vi "HW operation 3.vi"(1 "stop":bool) -> (0 "Numeric":dbl)   [LabVIEW 2018]
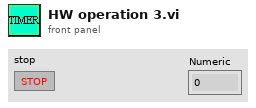
[diagram p1: front panel]
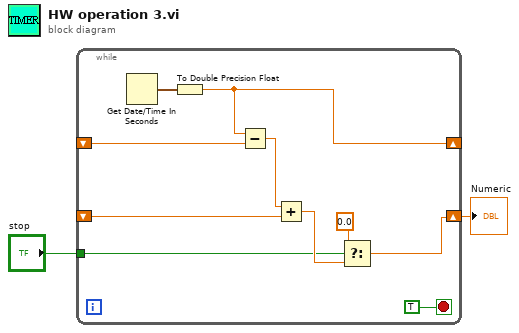
[diagram p0: block diagram]
diagram:
  n1 = while {
    shift-right: [w11] -> _
    shift-left: _ -> [w10]
    shift-right: [w3] -> w2
    shift-left: _ -> [w9]
    tunnel: "stop" -> [w4]
    stop <- TRUE stop-if-true
    n2 = Get Date/Time In Seconds() -> (seconds since 1Jan1904=w12:timestamp)
    n3 = To Double Precision Float(number=w12) -> (double precision float=w11:dbl)
    n4 = Subtract(x=w11, y=w10) -> (x-y=w8:dbl)
    n5 = Add(x=w8, y=w9) -> (x+y=w6:dbl)
    n6 = Select(t=0.0, s=w4, f=w6) -> (s? t:f=w3:dbl)
  }
  "Numeric" <- w2
